vi "ModBus test.vi"() -> ()   [LabVIEW 2016]
uses:
  <vilib>/NI/Modbus Library/API/Wrapper/Create TCP Master.vi
  <vilib>/NI/Modbus Library/API/Master/Modbus Master.lvclass
  <vilib>/NI/Modbus Library/API/Wrapper/API Main.lvlib
panel:
  out "coils":bool[](array[boolean])
  in  "coil to write":bool
  in  "starting coil address":u16
  out "*(type *) &x":string
  out "register values":u16[](array[numeric])=[18537, 8308, 26725, 29285, 8224, 8224, 8224, 8224, 8224, 8224, 8224, 8224, 8224, 8224, 8224, 8224, 8224, 8224, 8224, 8224, 8224, 8224, 8224, 8224, 8224, 8224, 8224, 8224, 8224, 8224, 8224, 8224, 8224, 8224, 8224, 8224, 8224, 8224, 8224, 8224, 8224, 8224, 8224, 8224, 8224, 8224, 8224, 8224, 8224, 8224, 8224, 8224, 8224, 8224, 8224, 8224, 8224, 8224, 8224, 8224, 8224, 8224, 8224, 8224, 8224, 8224, 0, 0, 0, 0, 0, 0, 0, 0, 0, 0, 0, 0, 0, 0, 0, 0, 0, 0, 0, 0, 0, 0, 0, 0, 0, 0, 0, 0, 0, 0, 0, 0, 0, 0, 0, 0, 0, 0, 0, 0, 0, 0, 0, 0, 0, 0, 0, 0, 0, 0, 0, 0, 0, 0, 0, 0, 0, 0, 0]
  in  "number of inputs":u16=125
  in  "starting holding address":u16=1200
  in  "address":string="192.168.1.20"
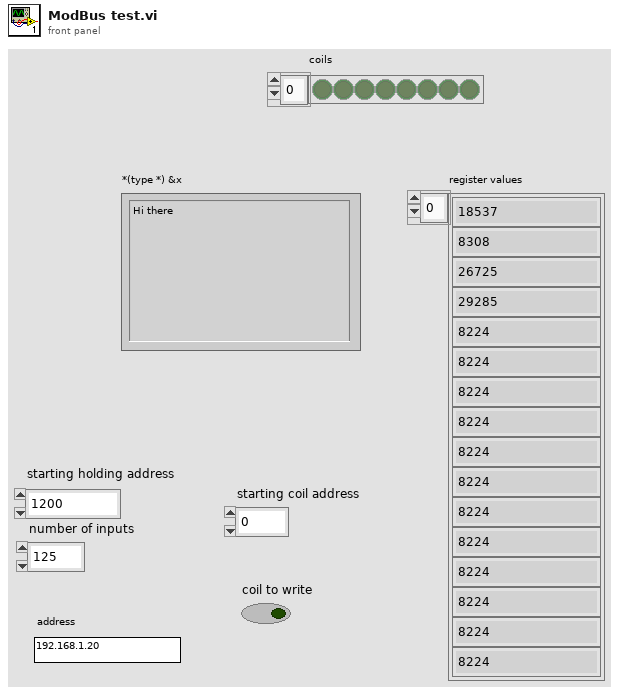
[diagram p1: front panel]
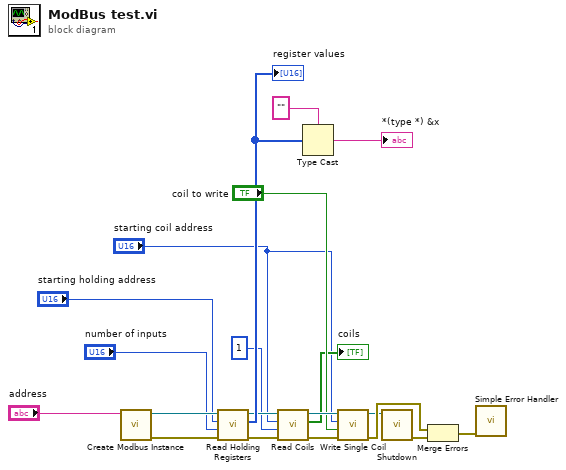
[diagram p0: block diagram]
diagram:
  n1 = call-poly <vilib>:"Create Modbus Instance.vi"("address"="address") -> ("error out"=w19:errorcluster, "TCP master instance"=w20:refnum<class "Modbus Master.lvclass">)  [unwired: 9 in]
  n2 = call-dynamic "Read Holding Registers.vi"("error in"=w19, "number of inputs"="number of inputs", "starting address"="starting holding address", "Modbus master in"=w20) -> ("error out"=w17:errorcluster, "register values"=w14:u16[], "Modbus master out"=w10:refnum<class "Modbus Master.lvclass">)  [unwired: 5 in]
  "register values" <- w14
  n3 = call-dynamic "Read Coils.vi"("error in"=w17, "number of inputs"=u16 1, "starting address"="starting coil address", "Modbus master in"=w10) -> ("error out"=w11:errorcluster, "coils"=→"coils":bool[], "Modbus master out"=w8:refnum<class "Modbus Master.lvclass">)  [unwired: 5 in]
  n4 = Type Cast(type="", x=w14) -> (*(type *) &x=→"*(type *) &x":string)
  n5 = call-dynamic "Write Single Coil.vi"("error in"=w11, "coil to write"="coil to write", "address"="starting coil address", "Modbus master in"=w8) -> ("error out"=w9:errorcluster, "Modbus master out"=w7:refnum<class "Modbus Master.lvclass">)  [unwired: 6 in]
  n6 = call-dynamic "Shutdown.vi"("Modbus master in"=w7) -> ("error out"=w18:errorcluster)  [unwired: 10 in]
  n7 = Merge Errors(w9, w18) -> (w16:errorcluster)
  n8 = call <vilib>:"Simple Error Handler.vi"("error in (no error)"=w16) -> ()  [unwired: 4 in, 5 out]
